vi "Example XYGraph Markers.vi"() -> ()   [LabVIEW 2020]
doc: "Graph extensions add the ability to have very capable and interactive markers placed on the graph. This GRAPH control has a custom palette icon for the \"cursor\" mode, which is replaced by graph extensions' markers mode.\n\nThis markers extension, has by default the the cursors extension included, which is activated automatically in the various other graph palette active tools. (like pan, zoom)."
uses:
  <vilib>/Analysis/1siggen.llb/Ramp Pattern by Samples.vi
  <vilib>/ptbypt/NI_PtbyPt.lvlib
  Graph Extensions.lvlib
  controls/commands.ctl
  <vilib>/Analysis/NI_AALBase.lvlib
panel:
  out "CursLoc":cluster{"X":dbl, "Y":dbl}
  out "XY Graph":cluster{dbl[], dbl[]}[](graph)
  # "Instructions:\n1. Run the VI, move the mouse over the graph.  \n2. The graph has to be in cursor (marker)mode to enable markers (the right hand button)\n3. Left click to follow instructions and place markers\n4. Right click to change the marker type, options or edit existing markers.\n5. Switch graph tools, to pan and markers will follow automatically."
  # "The cursor icon has been replaced for use\nwith the markers in graph extensions"
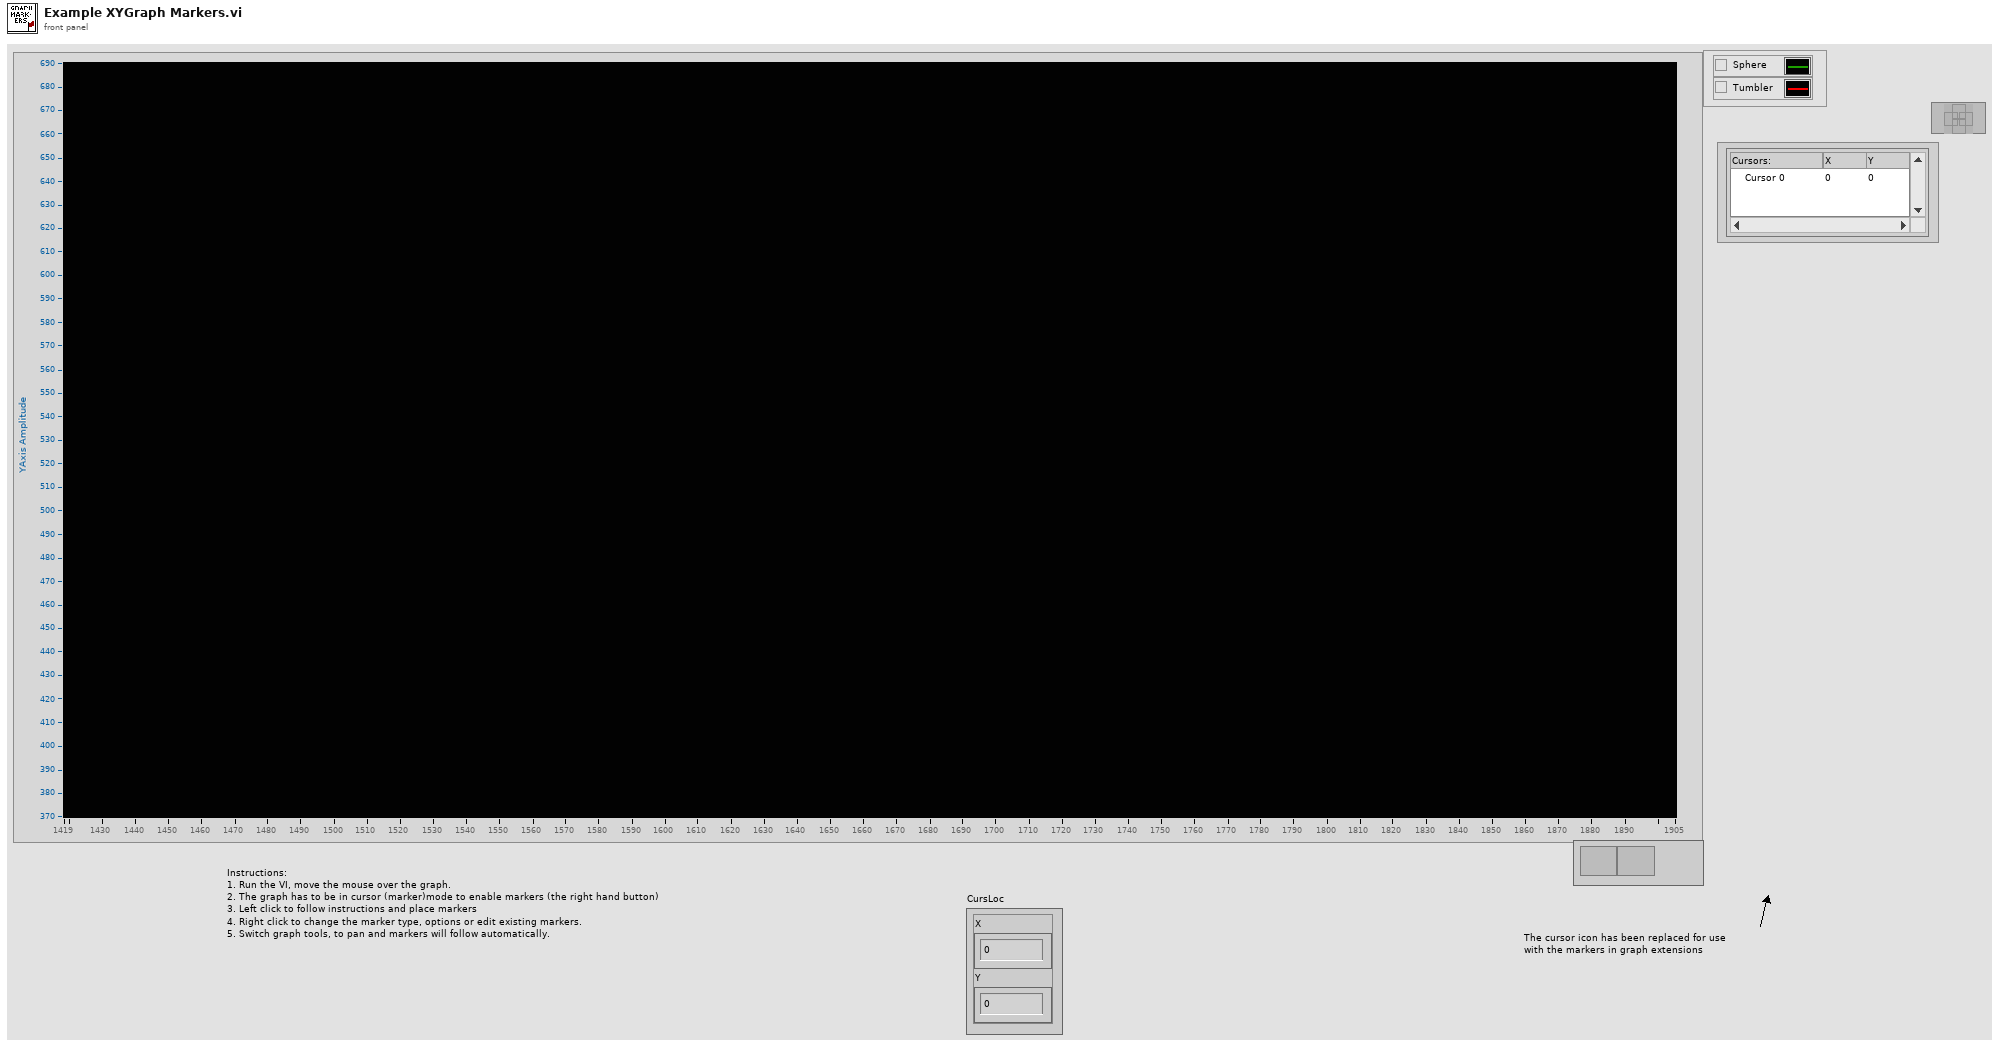
[diagram p1: front panel]
types:
  T1 = typedef "Graph Extensions.lvlib/commands.ctl" = enum16{"up", "options", "click", "move", "type", "redraw", "edited", "exit", "Mark"}
  T2 = typedef "LVPoint32TypeDef.ctl" = cluster{"Horizontal":i32, "Vertical":i32}
  T3 = typedef "Graph Extensions.lvlib/markerType.ctl" = enum16{"point", "arrow", "horiz", "vert", "vert range", "horiz range", "box"}
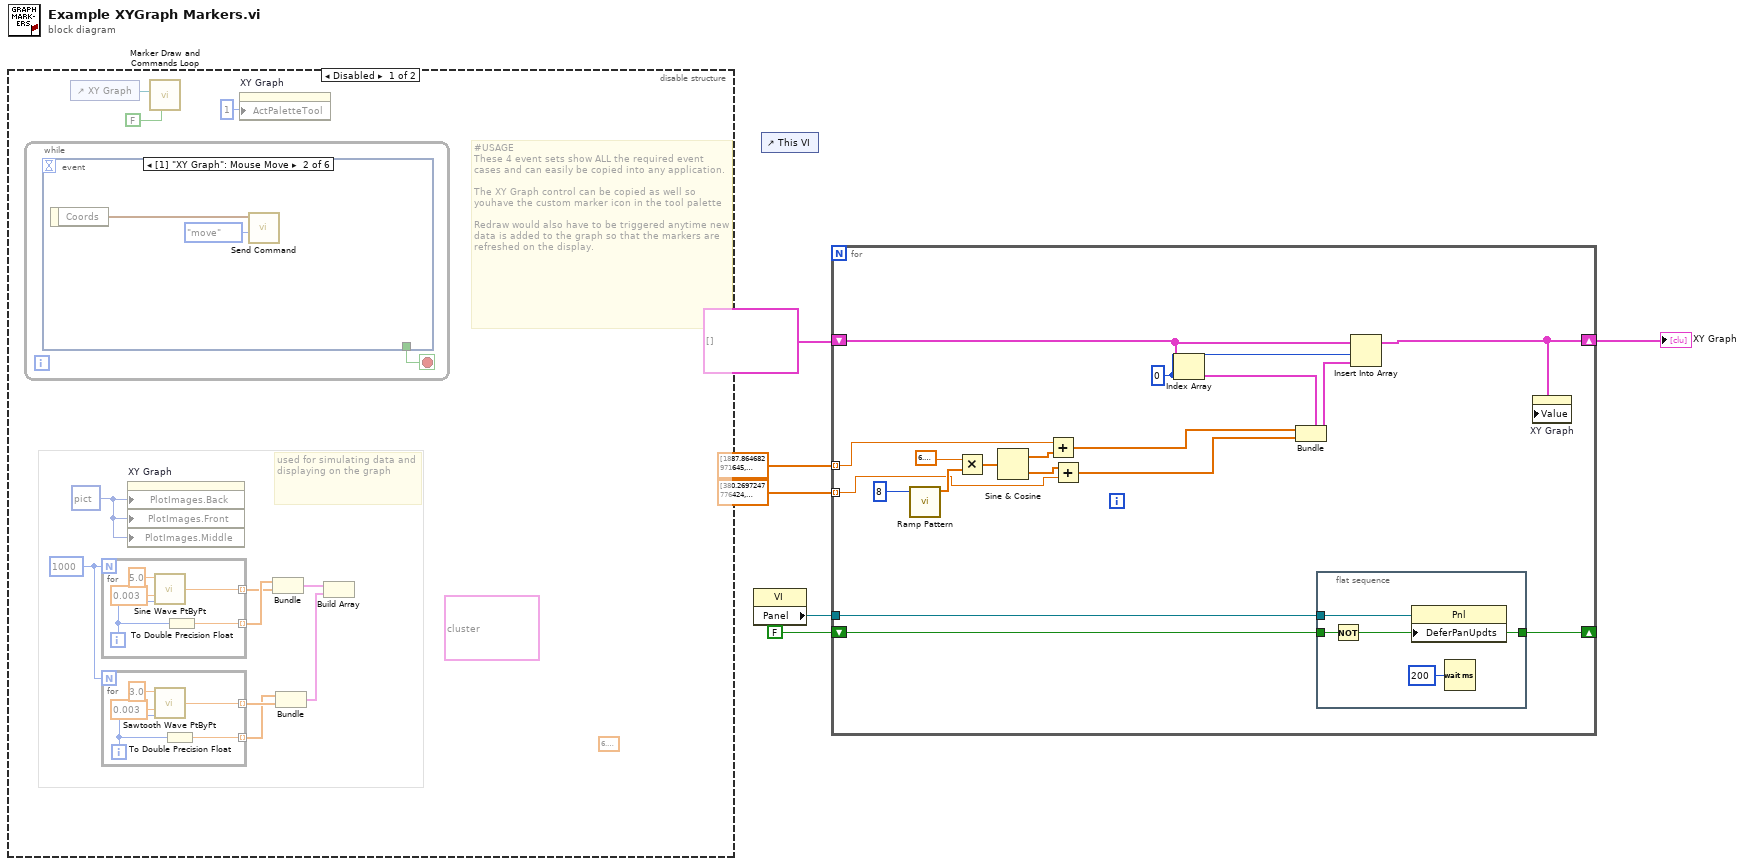
[diagram p0: block diagram]
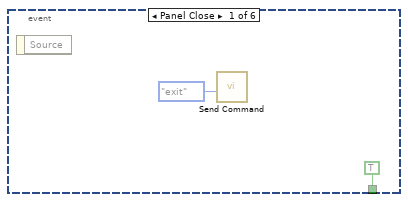
[diagram p2: hidden frame]
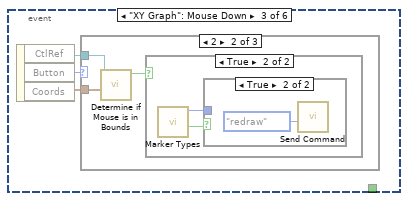
[diagram p3: hidden frame]
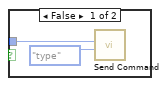
[diagram p6: hidden frame]
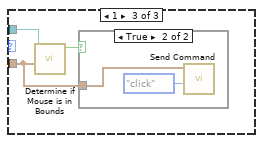
[diagram p7: hidden frame]
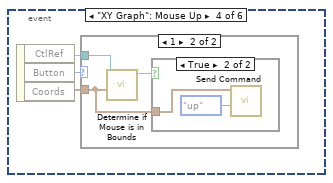
[diagram p9: hidden frame]
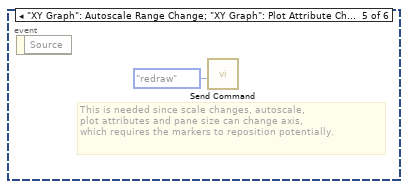
[diagram p12: hidden frame]
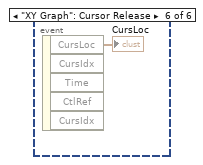
[diagram p13: hidden frame]
diagram:
  n1 = disable-structure shown="Disabled" {
    frame Disabled {
      (unwired) 6.283185307179586
      (unwired) cluster{dbl[], dbl[]}[] [{array[535 elements], array[535 elements]}, {array[535 elements], array[535 elements]}] ("XY Graph")
      w10 = picture data[5B] ("Plot Images:Back")
      w11 = 1000
      # "#USAGE\nThese 4 event sets show ALL the required event cases and can easily be copied into any application.\n\nThe XY Graph control can be copied as well so youhave the custom marker icon in the tool palette\n\nRedraw would also have to be triggered anytime new data is added to the graph so that the markers are refreshed on the display."
      # "used for simulating data and displaying on the graph"
      n2 = while {
        stop <- w18 stop-if-true
        n3 = event shown="[1] \"XY Graph\": Mouse Move" {
          selector: _ -> [_ _ _ _ _ _]
          dyn-events: _ -> [_ _ _ _ _ _]
          timeout: _ -> [_ _ _ _ _ _]
          tunnel: [TRUE _ _ _ _ _] -> w18
          event Panel Close {
            n4 = event-data() -> ()  [unwired: 1 in, 1 out]
            n5 = call "Send Command.vi"("cmd"=commands."exit") -> ()  [unwired: 11 in]
          }
          event "XY Graph": Mouse Move {
            n6 = event-data() -> ("Coords"=w22:T2)  [unwired: 1 in]
            n7 = call "Send Command.vi"("cmd"=commands."move", "Coords"=w22) -> ()  [unwired: 10 in]
          }
          event "XY Graph": Mouse Down {
            n8 = event-data() -> ("CtlRef"=w23:refnum<vi>, "Button"=w25:u16, "Coords"=w24:T2)  [unwired: 1 in]
            n9 = case shown="2" w25 {
              tunnel: w24 -> [_ w28 w35]
              tunnel: w23 -> [_ w27 w36]
              frame Default {
              }
              frame 2 {
                n10 = call "Determine if Mouse is in Bounds.vi"("Coords"=w28, "XYGraph in"=w27) -> ("In bounds?"=w26:bool)  [unwired: 9 in]
                n11 = case shown="True" w26 {
                  frame False {
                  }
                  frame True {
                    n12 = call "Marker Types.vi"() -> ("Close"=w30:bool, "Type"=w29:T3)  [unwired: 10 in]
                    n13 = case shown="True" w30 {
                      tunnel: w29 -> [w32 _]
                      frame False {
                        n14 = call "Send Command.vi"("cmd"=commands."type", "Type"=w32) -> ()  [unwired: 10 in]
                      }
                      frame True {
                        n15 = call "Send Command.vi"("cmd"=commands."redraw") -> ()  [unwired: 11 in]
                      }
                    }
                  }
                }
              }
              frame 1 {
                n16 = call "Determine if Mouse is in Bounds.vi"("Coords"=w35, "XYGraph in"=w36) -> ("In bounds?"=w34:bool)  [unwired: 9 in]
                n17 = case shown="True" w34 {
                  tunnel: w35 -> [_ w37]
                  frame False {
                  }
                  frame True {
                    n18 = call "Send Command.vi"("cmd"=commands."click", "Coords"=w37) -> ()  [unwired: 10 in]
                  }
                }
              }
            }
          }
          event "XY Graph": Mouse Up {
            n19 = event-data() -> ("CtlRef"=w39:refnum<vi>, "Button"=w41:u16, "Coords"=w40:T2)  [unwired: 1 in]
            n20 = case shown="1" w41 {
              tunnel: w40 -> [_ w43]
              tunnel: w39 -> [_ w44]
              frame Default {
              }
              frame 1 {
                n21 = call "Determine if Mouse is in Bounds.vi"("Coords"=w43, "XYGraph in"=w44) -> ("In bounds?"=w42:bool)  [unwired: 9 in]
                n22 = case shown="True" w42 {
                  tunnel: w43 -> [_ w45]
                  frame False {
                  }
                  frame True {
                    n23 = call "Send Command.vi"("cmd"=commands."up", "Coords"=w45) -> ()  [unwired: 10 in]
                  }
                }
              }
            }
          }
          event "XY Graph": Autoscale Range Change; "XY Graph": Plot Attribute Change; Pane Size {
            # "This is needed since scale changes, autoscale, \nplot attributes and pane size can change axis, \nwhich requires the markers to reposition potentially."
            n24 = event-data() -> ()  [unwired: 1 in, 1 out]
            n25 = call "Send Command.vi"("cmd"=commands."redraw") -> ()  [unwired: 11 in]
          }
          event "XY Graph": Cursor Release {
            n26 = event-data() -> ("CursLoc"=→"CursLoc":cluster{"X":dbl, "Y":dbl})  [unwired: 1 in, 4 out]
          }
        }
      }
      n27 = control-ref of="XY Graph"() -> (w8:refnum<vi>)
      n28 = for {
        N: w11 -> [_]
        tunnel: [w58] -> w16 mode=indexing
        tunnel: [w54] -> w17 mode=indexing
        i -> [w57]
        n29 = call <vilib>:"Sine Wave PtByPt.vi"("time"=w57, "frequency"=0.003, "amplitude"=5.0) -> ("sine wave"=w58:dbl)  [unwired: 1 in]
        n30 = To Double Precision Float(number=w57) -> (double precision float=w54:dbl)
      }
      n31 = for {
        N: w11 -> [_]
        tunnel: [w53] -> w14 mode=indexing
        tunnel: [w49] -> w13 mode=indexing
        i -> [w52]
        n32 = call <vilib>:"Sawtooth Wave PtByPt.vi"("time"=w52, "frequency"=0.003, "amplitude"=3.0) -> ("sawtooth wave"=w53:dbl)  [unwired: 1 in]
        n33 = To Double Precision Float(number=w52) -> (double precision float=w49:dbl)
      }
      n34 = property on="XY Graph" class="XYGraph (strict)"("PlotImages.Back"=w10, "PlotImages.Front"=w10, "PlotImages.Middle"=w10) -> ()  [unwired: 2 in, 2 out]
      n35 = call "Marker Draw and Commands Loop.vi"("Enable Cursors"=FALSE, "XY Graph"=w8) -> ()  [unwired: 10 in]
      n36 = property on="XY Graph" class="XYGraph (strict)"("ActPaletteTool"=1 ("Palette:Active Tool")) -> ()  [unwired: 2 in, 2 out]
      n37 = Bundle(w17, w16) -> (w15:cluster{dbl[], dbl[]})  [unwired: 1 in]
      n38 = Bundle(w13, w14) -> (w12:cluster{dbl[], dbl[]})  [unwired: 1 in]
      n39 = Build Array(w15, w12) -> ()  [unwired: 1 out]
    }
    frame Enabled {
    }
  }
  n40 = property class="VI"() -> ("Panel"=w2:refnum<vi>)  [unwired: 2 in, 2 out]
  n41 = control-ref of="This VI"() -> ()  [unwired: 1 out]
  n42 = for {
    tunnel: dbl[] [1887.864682971645, 1887.864682971645, 1878.784682971645, 1864.114682971645, 1876.864682971645, 1868.564682971644, 1887.864682971645, 1888.684682971645, 1876.864682971645, 1878.794682971644, 1876.664682971644, 1893.864682971645, 1893.864682971645, 1884.764682971645, 1871.554682971645, 1864.314682971644, 1893.874682971644, 1893.864682971645, 1893.864682971645, 1885.034682971645, 1893.864682971645, 1893.864682971645, 1880.534682971645, 1884.024682971645, 1879.584682971645, 1893.864682971645, 1893.864682971645, 1893.869664227359, 1888.059664227359, 1882.254682971645, 1876.249664227359, 1870.254682971645, 1864.249664227359, 1893.869664227359, 1893.869664227359, 1904.369664227359, 1898.949664227359, 1892.369664227359, 1886.719664227359, 1878.699664227359, 1884.43966422736, 1876.139664227359, 1853.264682971645, 1842.264682971645, 1859.374682971645, 1849.374682971644, 1839.374682971645, 1831.264682971645, 1820.264682971646, 1829.374682971644, 1819.374682971644, 1855.674682971644, 1833.744682971644, 1833.744682971644, 1809.264682971645, 1798.864682971645, 1809.374682971643, 1799.374682971644, 1789.374682971644, 1784.414682971643, 1775.874682971644, 1779.374682971645, 1769.374682971644, 1759.374682971644, 1766.144682971644, 1790.044682971644, 1795.874682971644, 1756.374682971644, 1746.604682971645, 1736.834682971644, 1749.374682971644, 1739.374682971645, 1727.054682971645, 1717.164682971644, 1706.854682971644, 1729.374682971643, 1721.404682971645, 1697.124682971644, 1687.124682971645, 1677.124682971645, 1667.124682971645, 1657.124682971645, 1752.614682971645, 1752.634682971644, 1735.034682971645, 1728.184682971645, 1661.654682971645, 1655.584682971644, 1858.124682971645, 1851.624682971644, 1814.374682971645, 1814.374682971645, 1827.624682971645, 1834.374682971644, 1821.114682971645, 1814.374682971645, 1854.369664227359, 1854.374682971643, 1854.364682971645, 1834.374682971644, 1834.994682971645, 1804.894682971644, 1794.794682971644, 1783.794682971644, 1766.904682971645, 1759.764682971645, 1768.944682971645, 1773.484682971645, 1768.634682971644, 1793.414682971643, 1858.254682971644, 1847.254682971645, 1852.249664227359, 1841.599664227359, 1813.364682971645, 1835.954682971644, 1830.299664227359, 1824.654682971645, 1818.999664227359, 1854.359664227359, 1854.359664227359, 1854.369664227359, 1834.989664227359, 1807.729664227359, 1796.579664227359, 1802.054682971645, 1791.054682971645, 1785.579664227359, 1780.054682971646, 1761.184682971645, 1769.054682971645, 1774.579664227359, 1763.579664227359, 1762.91966422736, 1757.944682971645, 1752.634682971644, 1742.844682971645, 1753.114682971645, 1754.614682971645, 1714.419664227359, 1716.034682971644, 1718.854682971645, 1754.114682971645, 1756.864682971645, 1748.654682971645, 1738.264682971645, 1727.844682971645, 1726.764682971645, 1717.914682971644, 1697.644682971645, 1699.794682971645, 1702.324682971645, 1695.834682971644, 1689.704682971645, 1674.854682971644, 1664.164682971645, 1704.439664227359, 1685.424682971645, 1704.574682971645, 1699.454682971644, 1668.594682971644, 1667.254682971645, 1665.954682971644, 1659.494682971645, 1749.864682971645, 1738.544682971644, 1736.054682971645, 1755.989664227359, 1748.349664227359, 1738.549664227359, 1738.549664227359, 1730.549664227359, 1719.549664227359, 1725.054682971645, 1714.054682971645, 1708.549664227359, 1755.779664227359, 1748.649664227359, 1738.269664227359, 1726.759664227359, 1727.839664227358, 1717.919664227359, 1698.634682971645, 1703.054682971646, 1687.804682971645, 1700.549664227359, 1689.749664227359, 1676.804682971645, 1662.694682971645, 1665.894682971646, 1678.749664227359, 1667.749664227359, 1661.169664227359, 1704.569664227358, 1699.459664227359, 1679.56966422736, 1663.679664227359, 1654.589664227359, 1667.989664227359, 1673.029664227359, 1904.369664227359, 1904.369664227359, 1904.369664227359, 1904.369664227359, 1904.369664227359, 1892.369664227359, 1885.039664227359, 1892.369664227359, 1892.369664227359, 1892.369664227359, 1904.369664227359, 1904.369664227359, 1904.369664227359, 1904.369664227359, 1892.369664227359, 1892.369664227359, 1883.079664227359, 1892.369664227359, 1864.31966422736, 1873.78966422736, 1892.369664227359, 1892.369664227359, 1882.369664227359, 1871.369664227359, 1902.65966422736, 1894.689664227359, 1886.649664227359, 1878.359664227359, 1864.11966422736, 1858.119664227359, 1851.619664227359, 1834.369664227358, 1834.369664227358, 1827.629664227359, 1821.109664227359, 1814.369664227359, 1856.08966422736, 1814.369664227359, 1814.369664227359, 1833.73966422736, 1793.409664227359, 1794.799664227358, 1783.799664227359, 1804.889664227359, 1773.489664227359, 1765.99966422736, 1761.039664227359, 1768.629664227358, 1795.85966422736, 1790.02966422736, 1768.939664227359, 1767.519664227359, 1860.36966422736, 1849.369664227359, 1839.369664227359, 1833.73966422736, 1829.369664227359, 1819.369664227359, 1853.259664227359, 1842.259664227359, 1831.259664227359, 1820.25966422736, 1809.369664227359, 1799.369664227359, 1789.369664227359, 1779.369664227359, 1769.369664227359, 1759.369664227359, 1809.259664227359, 1798.869664227359, 1784.419664227359, 1775.869664227359, 1766.149664227359, 1754.61966422736, 1754.61966422736, 1754.61966422736, 1736.589664227359, 1716.029664227359, 1718.85966422736, 1754.009664227359, 1757.369664227359, 1752.649664227359, 1747.369664227359, 1736.569664227358, 1728.169664227359, 1704.439664227359, 1686.10966422736, 1690.539664227359, 1695.839664227358, 1702.329664227359, 1696.179664227359, 1696.51966422736, 1693.109664227359, 1683.94966422736, 1677.73966422736, 1749.369664227359, 1739.36966422736, 1729.369664227359, 1721.409664227359, 1756.37966422736, 1746.599664227359, 1736.829664227359, 1727.059664227359, 1717.179664227359, 1706.389664227359, 1696.149664227359, 1685.639664227359, 1675.139664227359, 1664.629664227359, 1654.11966422736, 1641.724682971644, 1630.844682971644, 1620.204682971644, 1609.964682971645, 1599.504682971644, 1589.044682971645, 1578.594682971645, 1567.954682971644, 1558.154682971645, 1549.114682971645, 1567.954682971644, 1635.594682971644, 1645.594682971644, 1626.554682971644, 1616.554682971645, 1608.524682971644, 1652.434682971645, 1645.134682971645, 1616.954682971645, 1608.784682971645, 1600.484682971645, 1592.454682971645, 1593.964682971645, 1567.954682971644, 1592.454682971645, 1593.964682971645, 1600.624682971645, 1583.364682971645, 1573.994682971645, 1563.014682971645, 1552.754682971644, 1535.594682971645, 1527.444682971645, 1518.954682971645, 1509.084682971645, 1499.214682971645, 1518.954682971645, 1518.954682971645, 1489.354682971645, 1458.684682971645, 1446.104682971645, 1479.724682971645, 1469.954682971645, 1469.954682971645, 1543.454682971645, 1543.454682971645, 1518.954682971645, 1543.454682971645, 1543.454682971645, 1534.974682971645, 1526.504682971645, 1518.024682971645, 1498.404682971645, 1508.524682971645, 1494.454682971645, 1494.454682971645, 1469.954682971645, 1447.164682971645, 1494.454682971645, 1494.454682971645, 1487.424682971645, 1477.504682971645, 1616.954682971645, 1616.954682971645, 1647.724682971645, 1650.404682971645, 1645.044682971646, 1645.044682971646, 1571.614682971644, 1592.454682971645, 1586.574682971645, 1592.454682971645, 1592.454682971645, 1646.15966422736, 1638.484682971645, 1636.41966422736, 1629.384682971645, 1620.674682971644, 1602.054682971645, 1611.644682971645, 1604.879664227359, 1627.50966422736, 1618.95966422736, 1613.019664227359, 1646.709664227359, 1640.209664227359, 1618.95966422736, 1618.95966422736, 1592.454682971645, 1596.309664227359, 1589.859664227359, 1584.054682971645, 1575.814682971645, 1582.359664227359, 1573.489664227358, 1566.914682971645, 1571.229664227359, 1570.529664227359, 1565.064682971645, 1567.864682971644, 1568.869664227359, 1565.089664227359, 1558.654682971645, 1555.08966422736, 1549.484682971645, 1527.034682971645, 1518.954682971645, 1518.954682971645, 1519.194682971645, 1509.644682971645, 1542.454682971645, 1542.454682971645, 1534.874682971645, 1542.454682971645, 1499.614682971644, 1463.054682971645, 1493.454682971645, 1493.454682971645, 1455.814682971644, 1444.274682971645, 1518.954682971645, 1518.964682971645, 1538.494682971645, 1528.494682971644, 1521.479664227359, 1532.139664227359, 1518.954682971645, 1518.954682971645, 1511.659664227359, 1511.654682971645, 1503.609664227359, 1502.394682971645, 1490.084682971645, 1473.034682971644, 1486.469664227359, 1492.474682971645, 1482.304682971645, 1475.719664227359, 1456.99966422736, 1463.144682971645, 1455.084682971645, 1444.084682971644, 1443.999664227359, 1464.929664227359, 1433.514682971645, 1419.954682971645, 1419.954682971645, 1419.954682971645, 1438.824682971644, 1426.674682971645, 1419.954682971645, 1419.954682971645, 1429.804682971645, 1419.954682971645, 1419.954682971645, 1419.954682971645, 1419.954682971645, 1422.594682971644, 1422.594682971644, 1434.044682971645, 1421.954682971645, 1421.954682971645, 1421.954682971645, 1434.044682971645, 1434.044682971645, 1434.044682971645, 1434.044682971645, 1441.45966422736, 1643.45966422736, 1638.389664227359, 1626.82966422736, 1611.639664227359, 1602.979664227359, 1618.95966422736, 1594.45966422736, 1594.45966422736, 1549.229664227359, 1595.339664227359, 1566.609664227359, 1560.339664227359, 1548.919664227359, 1618.95966422736, 1618.95966422736, 1640.61966422736, 1629.819664227359, 1618.95966422736, 1608.649664227359, 1597.649664227359, 1586.649664227359, 1575.649664227359, 1564.649664227359, 1557.439664227359, 1550.269664227359, 1545.459664227359, 1539.769664227359, 1545.459664227359, 1520.959664227359, 1495.439664227359, 1496.45966422736, 1494.389664227359, 1493.429664227359, 1472.669664227359, 1469.879664227359, 1536.079664227359, 1528.479664227359, 1520.94966422736, 1520.94966422736, 1520.94966422736, 1508.659664227359, 1496.519664227359, 1484.219664227359, 1471.739664227358, 1459.269664227359, 1447.029664227359, 1441.45966422736, 1430.529664227359, 1419.529664227359, 1430.529664227359, 1426.27966422736, 1422.029664227359, 1422.029664227359, 1422.029664227359, 1422.029664227359, 1434.529664227359, 1422.029664227359] -> [w70] mode=indexing
    tunnel: dbl[] [380.2697247776424, 389.8997247776426, 376.0597247776425, 375.0497247776422, 386.9497247776417, 386.9497247776417, 400.539724777643, 410.4997247776419, 396.8297247776431, 413.9797247776425, 406.2697247776424, 424.3797247776422, 434.419724777643, 418.5997247776424, 417.969724777643, 421.949724777642, 454.499724777643, 444.4597247776421, 464.8097247776425, 465.9397247776426, 490.4597247776421, 501.419724777643, 473.7297247776433, 490.1497247776426, 483.0997247776424, 512.3897247776433, 523.3497247776425, 540.6859370087852, 531.5959370087849, 526.0997247776425, 531.5959370087849, 526.0997247776425, 531.5959370087849, 562.2259370087853, 551.2259370087844, 579.2459370087853, 570.8459370087844, 583.1059370087853, 570.5859370087853, 571.7659370087862, 583.1059370087853, 577.5159370087854, 374.8497247776425, 374.8497247776425, 386.9497247776417, 386.9497247776417, 386.9497247776417, 374.8497247776425, 374.8497247776425, 386.9497247776417, 386.9497247776417, 426.1297247776422, 412.6497247776426, 419.1497247776426, 374.8497247776425, 375.1397247776423, 386.9497247776417, 386.9497247776417, 386.9497247776417, 376.0497247776431, 374.9797247776424, 386.9497247776417, 386.9497247776417, 386.9497247776417, 375.6997247776417, 414.7297247776426, 417.5997247776424, 375.6997247776417, 375.6997247776417, 375.6997247776417, 386.9497247776417, 386.9497247776417, 375.6997247776417, 375.2997247776423, 377.2897247776431, 386.9497247776417, 386.9497247776417, 374.9797247776424, 374.8497247776425, 374.8497247776425, 374.8497247776425, 374.8497247776425, 420.3397247776421, 427.3397247776421, 425.5797247776428, 420.5497247776421, 416.7497247776419, 421.1297247776423, 451.6797247776421, 451.6797247776421, 429.7397247776419, 440.1097247776426, 458.1897247776425, 462.1097247776425, 454.3897247776424, 450.469724777643, 473.475937008786, 499.8797247776422, 493.3097247776417, 472.0097247776424, 481.909724777643, 455.9897247776416, 460.3597247776425, 460.3597247776425, 430.579724777643, 429.5597247776425, 441.3897247776424, 458.8897247776433, 452.3797247776421, 472.0297247776426, 526.0997247776425, 526.0997247776425, 531.5959370087849, 531.5959370087849, 522.0797247776419, 526.0997247776425, 531.5959370087849, 526.0997247776425, 531.5959370087849, 557.8159370087853, 564.3159370087853, 584.2159370087854, 575.7759370087853, 531.5959370087849, 531.5959370087849, 526.0997247776425, 526.0997247776425, 531.5959370087849, 526.0997247776425, 518.409724777643, 526.0997247776425, 531.5959370087849, 531.5959370087849, 579.3459370087853, 441.3897247776424, 435.4897247776425, 429.3897247776424, 449.7497247776419, 460.6997247776426, 430.3159370087853, 451.5097247776422, 457.3597247776425, 468.199724777643, 476.759724777643, 474.6697247776421, 478.2997247776421, 475.3697247776419, 491.2397247776428, 487.079724777642, 428.9997247776419, 439.9297247776423, 447.789724777643, 450.449724777643, 459.169724777643, 465.9897247776416, 464.959724777643, 468.9859370087864, 467.8097247776426, 491.4397247776426, 487.4297247776421, 475.0397247776417, 485.0597247776426, 494.799724777643, 502.4397247776426, 517.0197247776424, 515.6397247776426, 526.3497247776425, 537.885937008785, 544.3459370087849, 542.055937008785, 532.3559370087852, 531.6659370087846, 531.6659370087846, 526.3497247776425, 526.3497247776425, 531.6659370087846, 581.1859370087863, 583.0259370087853, 579.3959370087852, 566.4559370087844, 582.3259370087852, 570.6159370087853, 518.2797247776426, 526.3497247776425, 516.3797247776422, 539.2059370087856, 541.3159370087853, 516.3797247776422, 509.4097247776427, 516.3797247776422, 541.3159370087853, 541.3159370087853, 546.6259370087852, 566.2559370087852, 570.2659370087854, 583.8659370087864, 557.1859370087853, 551.9259370087864, 566.7559370087852, 575.9659370087844, 599.4559370087854, 589.3559370087864, 609.5559370087844, 619.6659370087852, 629.7659370087845, 593.8459370087853, 591.7559370087844, 603.5159370087853, 613.1959370087843, 624.1759370087852, 639.8759370087852, 649.9759370087854, 660.0759370087853, 670.1859370087843, 642.7959370087844, 633.4859370087845, 640.8759370087843, 652.1159370087852, 635.7459370087854, 638.9559370087843, 661.4259370087843, 670.4859370087863, 670.7359370087845, 670.7359370087845, 680.2759370087853, 681.7459370087854, 681.7459370087854, 681.3659370087864, 682.6359370087843, 606.0159370087854, 606.0159370087854, 595.5859370087853, 585.6759370087852, 599.5059370087845, 603.2959370087852, 607.2159370087845, 631.7759370087854, 627.9559370087854, 617.5859370087843, 638.5459370087852, 585.6659370087843, 597.3359370087844, 597.3359370087844, 601.7059370087854, 598.7959370087844, 594.0359370087853, 587.7559370087854, 605.3059370087853, 640.0959370087844, 642.9659370087845, 616.3059370087853, 627.2159370087845, 670.7359370087845, 670.7359370087845, 670.7359370087845, 645.0459370087844, 670.7359370087845, 670.7359370087845, 682.8459370087853, 682.8459370087853, 682.8459370087853, 682.8459370087853, 670.7359370087845, 670.7359370087845, 670.7359370087845, 670.7359370087845, 670.7359370087845, 670.7359370087845, 682.8459370087853, 682.5459370087844, 681.6359370087844, 682.7159370087854, 681.9859370087854, 589.4559370087854, 608.8959370087852, 599.1659370087843, 597.5559370087864, 606.1859370087863, 600.3259370087844, 619.4259370087852, 628.1759370087852, 634.2359370087854, 628.1759370087852, 630.2459370087854, 637.3559370087853, 588.7059370087842, 591.7559370087844, 601.2759370087863, 607.2359370087854, 609.8959370087852, 614.3059370087844, 621.3659370087864, 631.3059370087853, 636.4359370087843, 639.9959370087844, 670.7359370087845, 670.7359370087845, 670.7359370087845, 670.7359370087845, 681.9859370087854, 681.9859370087854, 681.9859370087854, 681.9859370087854, 682.3959370087842, 680.3359370087853, 682.7159370087854, 682.7459370087853, 682.7459370087853, 682.7459370087853, 682.7459370087853, 374.8497247776425, 376.9097247776426, 377.0897247776429, 374.9497247776417, 374.9497247776417, 374.9497247776417, 374.9497247776417, 374.8697247776428, 374.9497247776417, 376.2897247776419, 404.0197247776424, 419.1697247776422, 421.0697247776427, 416.4697247776423, 416.4697247776423, 420.5697247776424, 456.7297247776425, 458.1397247776421, 470.5997247776424, 465.8797247776431, 424.3697247776419, 428.1597247776427, 438.4897247776416, 414.0197247776423, 456.4497247776426, 448.039724777643, 461.1697247776421, 461.6997247776427, 466.449724777643, 465.789724777643, 461.8297247776417, 376.9297247776425, 374.9797247776424, 374.9497247776417, 374.9497247776417, 374.9497247776417, 384.8697247776429, 404.0197247776424, 375.5397247776431, 375.2597247776422, 374.9497247776417, 377.709724777642, 381.8797247776423, 404.0197247776424, 428.1597247776427, 437.5297247776427, 414.0197247776423, 447.0797247776419, 456.4497247776426, 461.3497247776425, 466.2397247776428, 471.1397247776432, 461.789724777643, 465.7597247776424, 436.8097247776424, 428.1597247776427, 413.9697247776423, 425.6897247776426, 445.4297247776422, 454.0497247776421, 461.1597247776427, 466.0097247776421, 477.5997247776425, 494.3897247776424, 515.5597247776434, 507.6897247776425, 523.4297247776433, 534.4297247776426, 500.9997247776431, 513.039724777643, 509.6397247776423, 531.8997247776433, 522.4697247776421, 548.6559370087843, 542.6297247776422, 549.3859370087853, 547.8597247776424, 552.7797247776423, 545.7097247776424, 551.0997247776425, 551.7659370087852, 554.4959370087853, 561.4159370087852, 557.5559370087863, 598.4459370087852, 598.4459370087852, 571.9159370087843, 582.3059370087853, 541.329724777643, 548.9759370087853, 547.9859370087864, 545.7497247776424, 550.4797247776424, 552.1459370087853, 558.6759370087844, 558.8797247776424, 566.1859370087864, 577.6359370087853, 581.1497247776424, 571.7097247776424, 586.5559370087853, 591.8359370087853, 588.8297247776424, 596.4359370087852, 593.3597247776424, 503.549724777643, 480.3897247776424, 489.6797247776434, 499.0297247776427, 503.7797247776426, 519.6797247776434, 513.039724777643, 508.079724777642, 535.8297247776416, 509.7197247776424, 503.4797247776425, 518.409724777643, 534.2797247776417, 507.1497247776417, 513.2797247776427, 555.4697247776434, 564.9597247776425, 593.6097247776412, 589.0197247776425, 591.3459370087853, 594.0759370087844, 583.5397247776425, 574.3097247776433, 593.1959370087843, 586.8997247776433, 599.1459370087864, 592.7897247776424, 541.5997247776414, 584.9697247776423, 596.1659370087852, 594.0397247776425, 590.8897247776423, 591.6359370087852, 582.5159370087853, 580.1497247776423, 576.2197247776423, 576.0197247776434, 582.5159370087853, 586.3859370087852, 374.9497247776417, 374.9497247776417, 396.949724777642, 385.9497247776426, 429.6797247776424, 416.3497247776424, 407.9497247776425, 424.7397247776418, 433.9897247776429, 446.7397247776427, 435.7397247776424, 471.5897247776421, 457.7397247776425, 489.0097247776431, 477.6797247776421, 518.429724777643, 508.3297247776421, 498.2397247776416, 518.429724777643, 531.4297247776424, 557.4297247776424, 544.4297247776422, 570.4297247776423, 591.7459370087853, 629.7359370087853, 633.8059370087853, 642.1159370087853, 639.6559370087864, 634.6559370087851, 646.4759370087854, 608.9459370087852, 618.5059370087854, 600.2559370087854, 629.2759370087853, 640.2259370087845, 638.5059370087853, 629.2359370087853, 657.4759370087853, 668.4759370087833, 681.9659370087854, 680.4359370087843, 679.4759370087854, 682.7459370087853, 682.7459370087853, 682.7459370087853, 682.7459370087853, 682.7459370087853, 681.2459370087845, 681.7959370087852, 606.9459370087843, 600.2859370087853, 623.7359370087854, 648.3859370087852, 610.8959370087842, 601.4459370087852, 620.3359370087853, 628.2759370087854, 647.1659370087852, 641.2959370087844, 680.3959370087852, 679.6659370087852, 669.7359370087854, 658.5359370087854, 680.9359370087843, 685.7359370087854, 682.7459370087853, 680.5259370087845, 681.1159370087852, 680.2159370087854, 682.7459370087853, 606.9159370087843, 608.1859370087852, 608.1859370087852, 619.1859370087852, 628.3959370087853, 637.6059370087853, 648.8859370087852, 660.1759370087852, 671.4559370087843, 682.7459370087853, 682.7459370087853] -> [w69] mode=indexing
    shift-right: [w66] -> w3
    shift-left: cluster{dbl[], dbl[]}[] [] -> [w68]
    tunnel: w2 -> [w63]
    shift-right: [w64] -> _
    shift-left: FALSE ("Defer Panel Updates") -> [w65]
    w67 = 0 ("index")
    n43 = call-poly <vilib>:"Ramp Pattern.vi"("samples"=8) -> ("Ramp Pattern"=w74:dbl[])  [unwired: 9 in, 1 out]
    n44 = Multiply(x=6.283185307179586, y=w74) -> (x*y=w73:dbl[])
    n45 = Sine & Cosine(0:w73) -> (1:w72:dbl[], 2:w71:dbl[])
    n46 = Add(x=w70, y=w72) -> (x+y=w60:dbl[])
    n47 = Add(x=w71, y=w69) -> (x+y=w59:dbl[])
    n48 = Index Array(array=w68, index=w67) -> (element=w62:cluster{dbl[], dbl[]})
    n49 = Bundle(cluster=w62, w60, w59) -> (w61:cluster{dbl[], dbl[]})
    n50 = flat-sequence {
      tunnel: w65 -> [w79]
      tunnel: [w78] -> w64
      tunnel: w63 -> [w77]
      frame #0 {
        n51 = Not(x=w79) -> (.not. x?=w78:bool)
        n52 = property class="Pnl"(reference=w77, "DeferPanUpdts"=w78) -> ()  [unwired: 1 in, 2 out]
        n53 = Wait (ms)(milliseconds to wait=u32 200) -> ()  [unwired: 1 out]
      }
    }
    n54 = Insert Into Array(array=w68, index=w67, new element=w61) -> (w66:cluster{dbl[], dbl[]}[])
    n55 = property on="XY Graph" class="XYGraph (strict)"("Value"=w66) -> ()  [unwired: 2 in, 2 out]
  }
  "XY Graph" <- w3
